vi "Update WayPt Angles.vi"(6 "Min R":dbl, 8 "Blends In":T1[](array[typedef]), 9 "Index":i32, 10 "Waypoints in":cluster{"x":dbl, "y":dbl, "th":dbl}[](array[cluster]), 11 "th":dbl) -> (1 "Blends Out":T1[](array[typedef]), 3 "Waypoints out":cluster{"x":dbl, "y":dbl, "th":dbl}[](array[cluster]))   [LabVIEW 2018]
uses:
  BlendType.ctl
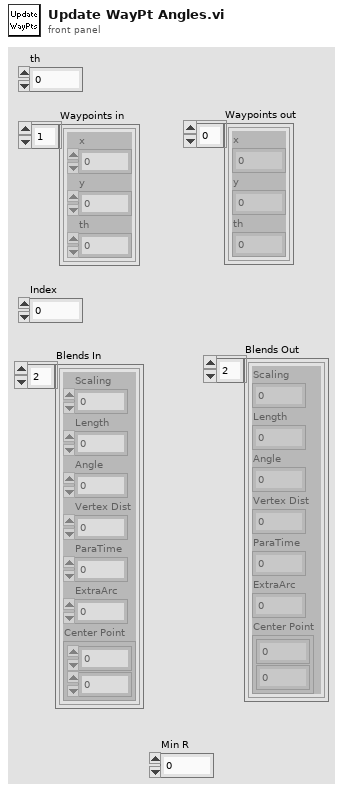
[diagram p1: front panel]
types:
  T1 = typedef "BlendType.ctl" = cluster{"Scaling":dbl, "Length":dbl, "Angle":dbl, "Vertex Dist":dbl, "ParaTime":dbl, "ExtraArc":dbl, "Center Point":cluster{dbl, dbl}}
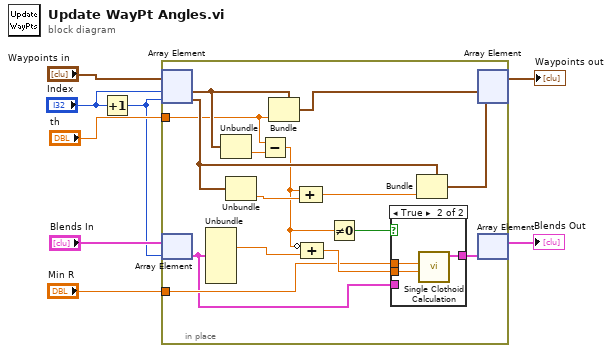
[diagram p0: block diagram]
diagram:
  n1 = Increment(x="Index") -> (x+1=w2:i32)
  n2 = in-place {
    in-place-border: "th" -> [w16]
    in-place-border: "Min R" -> [w13]
    n3 = in-place-array #1("Waypoints in", "Index", w2) -> (w19:cluster{"x":dbl, "y":dbl, "th":dbl}, w22:cluster{"x":dbl, "y":dbl, "th":dbl})
    n4 = in-place-array #2("Blends In", w2) -> (w11:T1)
    n5 = Unbundle(w11) -> ("Angle"=w15:dbl)  [unwired: 6 out]
    n6 = Unbundle(w19) -> ("th"=w17:dbl)  [unwired: 2 out]
    n7 = Unbundle(w22) -> ("th"=w20:dbl)  [unwired: 2 out]
    n8 = Subtract(x=w16, y=w17) -> (x-y=w10:dbl)
    n9 = Bundle(cluster=w19, "th"=w16) -> (w23:cluster{"x":dbl, "y":dbl, "th":dbl})  [unwired: 2 in]
    n10 = Compound Arithmetic op=ADD(w10, w20) -> (w18:dbl)
    n11 = Compound Arithmetic op=ADD(invert w10, w15) -> (w14:dbl)
    n12 = Not Equal To 0?(x=w10) -> (x != 0?=w9:bool)
    n13 = case shown="True" w9 {
      tunnel: w14 -> [_ w27]
      tunnel: w13 -> [_ w26]
      tunnel: [w24 w25] -> w12
      tunnel: w11 -> [w24 _]
      frame False {
      }
      frame True {
        n14 = call "Single Clothoid Calculation.vi"("Angle"=w27, "Min R"=w26) -> ("Zeroes out"=w25:T1)  [unwired: 9 in]
      }
    }
    n15 = Bundle(cluster=w22, "th"=w18) -> (w21:cluster{"x":dbl, "y":dbl, "th":dbl})  [unwired: 2 in]
    n16 = in-place-array #1(w23, w21) -> (→"Waypoints out":cluster{"x":dbl, "y":dbl, "th":dbl}[])  [unwired: 2 out]
    n17 = in-place-array #2(w12) -> (→"Blends Out":T1[])  [unwired: 1 out]
  }
